vi "Configure Power Measurement Single Parameter Set.vi"(0 "VISA resource name":refnum<visa-resource-name>, 1 "Bandwidth (300kHz)":dbl=300000.0 format="%#.9p", 2 "Measurement Length (450.0E-6)":dbl=0.00045 format="%^.3e", 5 "Instance (1)":i32=1, 7 "Parameter List (0)":i32, 9 "Filter Type (Gauss)":i32(ring) items=["Gauss", "Bandpass", "WCDMA", "CDMA", "TDSCdma"], 11 "error in (no error)":errorcluster, 12 "Step Length (576.9230769E-6)":dbl=0.0005769230769 format="%^.3e", 13 "Offset (50.0E-6)":dbl=5e-05 format="%^.3e") -> (4 "VISA resource name out":refnum<visa-resource-name>, 15 "error out":errorcluster)   [LabVIEW 2015, in "Rohde&Schwarz CMXP GPRF.lvlib"]
doc: "This VI sets a combination of measurement control settings. The \"Parameter List\" contains 32 possibly different parameter sets which you may assign to the individual measurement steps in list mode.\n\nAttributes:\nRSCMXPGPRF_ATTR_POWER_MEASUREMENT_PARAMETER_SET_FILTER_TYPE\nRSCMXPGPRF_ATTR_POWER_MEASUREMENT_PARAMETER_SET_GAUSS_BW\nRSCMXPGPRF_ATTR_POWER_MEASUREMENT_PARAMETER_SET_BANDPASS_BW\nRSCMXPGPRF_ATTR_POWER_MEASUREMENT_PARAMETER_SET_STEP_LENGTH\nRSCMXPGPRF_ATTR_POWER_MEASUREMENT_PARAMETER_SET_MEASUREMENT_LENGTH\nRSCMXPGPRF_ATTR_POWER_MEASUREMENT_PARAMETER_SET_OFFSET\n\nRemote-control commands:\nCONFigure:GPRF:MEAS<i>:POWer:PSET:FILTer:TYPE\nCONFigure:GPRF:MEAS<i>:POWer:PSET:FILTer:GAUSs:BWIDth\nCONFigure:GPRF:MEAS<i>:POWer:PSET:FILTer:BANDpass:BWIDth\nCONFigure:GPRF:MEAS<i>:POWer:PSET:SLENgth\nCONFigure:GPRF:MEAS<i>:POWer:PSET:MLENgth\nTRIGger:GPRF:MEAS<i>:POWer:PSET:OFFSet"
uses:
  <instrlib>/Rohde&Schwarz CMXP GPRF/Rohde&Schwarz CMXP GPRF.lvlib
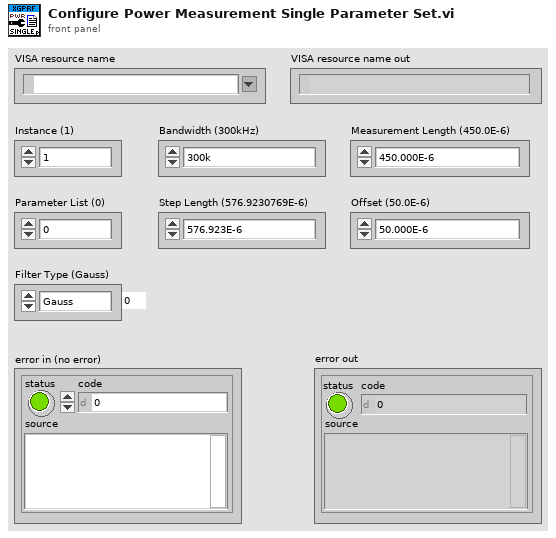
[diagram p1: front panel]
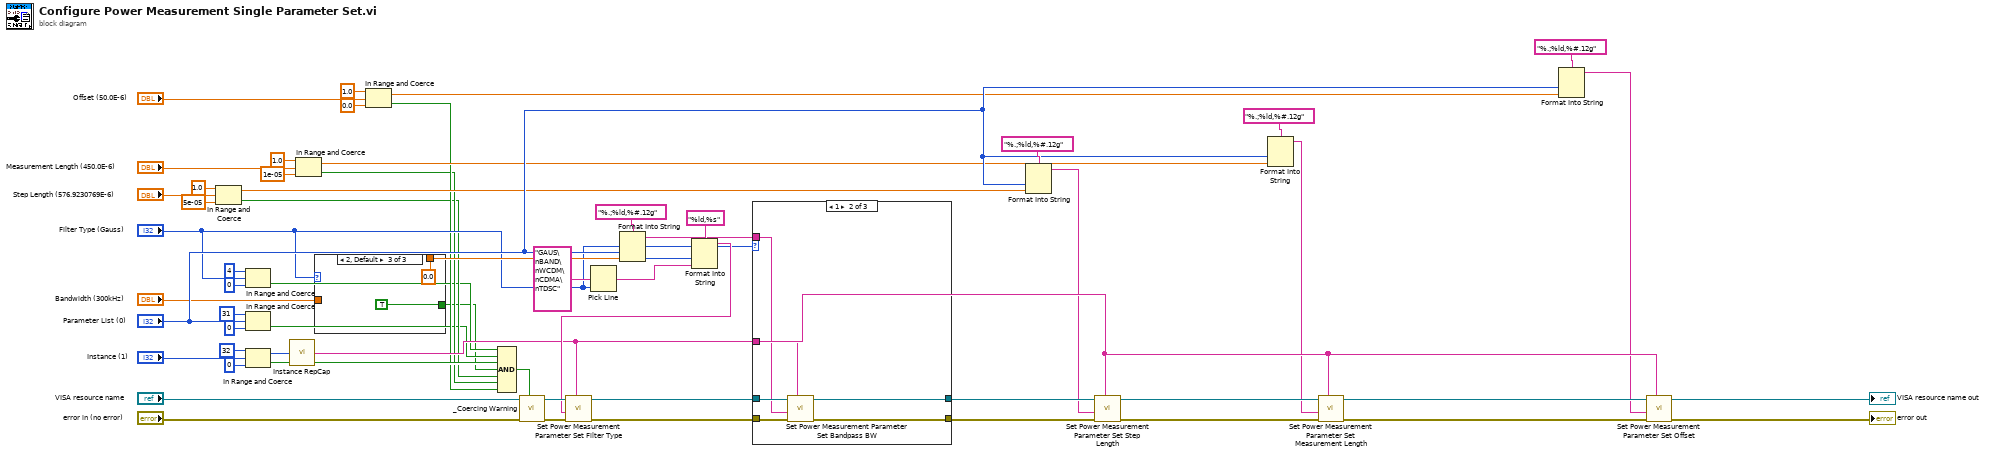
[diagram p0: block diagram]
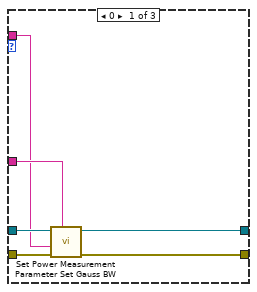
[diagram p2: hidden frame]
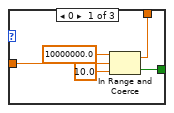
[diagram p4: hidden frame]
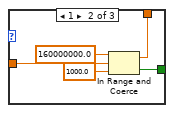
[diagram p5: hidden frame]
diagram:
  n1 = In Range and Coerce(upper limit=1.0, x="Step Length (576.9230769E-6)", lower limit=5e-05) -> (coerced(x)=w12:dbl, In Range?=w7:bool)
  n2 = In Range and Coerce(upper limit=4, x="Filter Type (Gauss)", lower limit=0) -> (In Range?=w5:bool)  [unwired: 1 out]
  n3 = In Range and Coerce(upper limit=31, x="Parameter List (0)", lower limit=0) -> (In Range?=w6:bool)  [unwired: 1 out]
  n4 = In Range and Coerce(upper limit=32, x="Instance (1)", lower limit=0) -> (coerced(x)=w31:i32, In Range?=w38:bool)
  n5 = call <instrlib>:"Instance RepCap.vi"("Instance in"=w31) -> ("Instance out"=w19:string)
  n6 = In Range and Coerce(upper limit=1.0, x="Measurement Length (450.0E-6)", lower limit=1e-05) -> (coerced(x)=w11:dbl, In Range?=w8:bool)
  n7 = case shown="2, Default" "Filter Type (Gauss)" {
    tunnel: "Bandwidth (300kHz)" -> [w62 w67 _]
    tunnel: [w61 w66 TRUE] -> w1
    tunnel: [w60 w65 0.0 ("upper limit")] -> w17
    frame 0 {
      n8 = In Range and Coerce(upper limit=10000000.0, x=w62, lower limit=10.0) -> (coerced(x)=w60:dbl, In Range?=w61:bool)
    }
    frame 1 {
      n9 = In Range and Coerce(upper limit=160000000.0, x=w67, lower limit=1000.0) -> (coerced(x)=w65:dbl, In Range?=w66:bool)
    }
    frame 2, Default {
    }
  }
  n10 = In Range and Coerce(upper limit=1.0, x="Offset (50.0E-6)", lower limit=0.0) -> (coerced(x)=w10:dbl, In Range?=w9:bool)
  n11 = Compound Arithmetic op=AND(w5, w6, w38, w1, w7, w8, w9) -> (w49:bool)
  n12 = call <instrlib>:"_Coercing Warning.vi"("In Range?"=w49, "error in (no error)"="error in (no error)", "VISA resource name"="VISA resource name") -> ("error out"=w36:errorcluster, "VISA resource name out"=w35:refnum<visa-resource-name>)  [unwired: 7 in]
  n13 = Pick Line(multi-line string="GAUS\nBAND\nWCDM\nCDMA\nTDSC", line index="Filter Type (Gauss)") -> (output string=w37:string)  [unwired: 1 in]
  n14 = Format Into String(format string="%.;%ld,%#.12g", "Parameter List (0)", w17) -> (resulting string=w29:string)  [unwired: 2 in, 1 out]
  n15 = Format Into String(format string="%ld,%s", "Parameter List (0)", w37) -> (resulting string=w32:string)  [unwired: 2 in, 1 out]
  n16 = call "Set Power Measurement Parameter Set Filter Type"("Repeated Capabilities"=w19, "error in (no error)"=w36, "Power Measurement Parameter Set Filter Type ()"=w32, "instrument handle"=w35) -> ("error out"=w34:errorcluster, "instrument handle out"=w33:refnum<visa-resource-name>)  [unwired: 6 in]
  n17 = case shown="1" "Filter Type (Gauss)" {
    tunnel: [w76 w82 w84] -> w28
    tunnel: [w75 w81 w85] -> w27
    tunnel: w34 -> [w77 w83 w84]
    tunnel: w33 -> [w74 w80 w85]
    tunnel: w29 -> [w72 w78 _]
    tunnel: w19 -> [w73 w79 _]
    frame 0 {
      n18 = call "Set Power Measurement Parameter Set Gauss BW"("Repeated Capabilities"=w73, "error in (no error)"=w77, "Power Measurement Parameter Set Gauss BW ()"=w72, "instrument handle"=w74) -> ("error out"=w76:errorcluster, "instrument handle out"=w75:refnum<visa-resource-name>)  [unwired: 6 in]
    }
    frame 1 {
      n19 = call "Set Power Measurement Parameter Set Bandpass BW"("Repeated Capabilities"=w79, "error in (no error)"=w83, "Power Measurement Parameter Set Bandpass BW ()"=w78, "instrument handle"=w80) -> ("error out"=w82:errorcluster, "instrument handle out"=w81:refnum<visa-resource-name>)  [unwired: 6 in]
    }
    frame Default {
    }
  }
  n20 = Format Into String(format string="%.;%ld,%#.12g", "Parameter List (0)", w12) -> (resulting string=w2:string)  [unwired: 2 in, 1 out]
  n21 = call "Set Power Measurement Parameter Set Step Length"("Repeated Capabilities"=w19, "error in (no error)"=w28, "Power Measurement Parameter Set Step Length ()"=w2, "instrument handle"=w27) -> ("error out"=w26:errorcluster, "instrument handle out"=w25:refnum<visa-resource-name>)  [unwired: 6 in]
  n22 = Format Into String(format string="%.;%ld,%#.12g", "Parameter List (0)", w11) -> (resulting string=w3:string)  [unwired: 2 in, 1 out]
  n23 = call "Set Power Measurement Parameter Set Measurement Length"("Repeated Capabilities"=w19, "error in (no error)"=w26, "Power Measurement Parameter Set Measurement Length ()"=w3, "instrument handle"=w25) -> ("error out"=w23:errorcluster, "instrument handle out"=w22:refnum<visa-resource-name>)  [unwired: 6 in]
  n24 = Format Into String(format string="%.;%ld,%#.12g", "Parameter List (0)", w10) -> (resulting string=w4:string)  [unwired: 2 in, 1 out]
  n25 = call "Set Power Measurement Parameter Set Offset"("Repeated Capabilities"=w19, "error in (no error)"=w23, "Power Measurement Parameter Set Offset ()"=w4, "instrument handle"=w22) -> ("error out"=→"error out":errorcluster, "instrument handle out"=→"VISA resource name out":refnum<visa-resource-name>)  [unwired: 6 in]
